vi "Init.vi"(8 "error in (no error)":errorcluster, 11 "DtoA in":refnum<class "Wavepond.lvclass">) -> (0 "error out":errorcluster, 3 "DtoA out":refnum<class "Wavepond.lvclass">)   [LabVIEW 2015, in "Wavepond.lvclass"]
uses:
  Wavepond.lvclass
  External Clock.lvclass
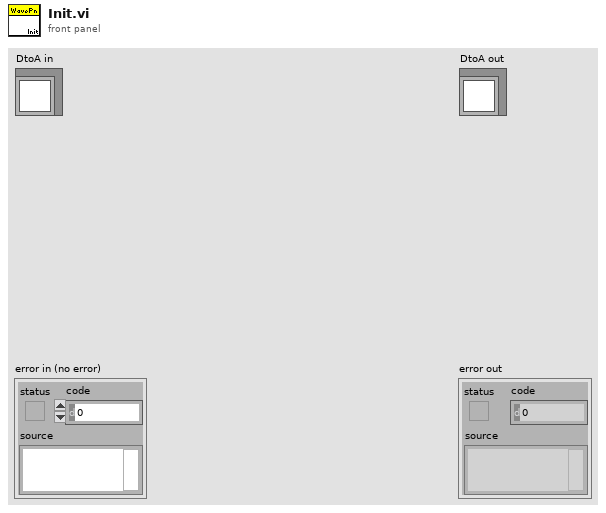
[diagram p1: front panel]
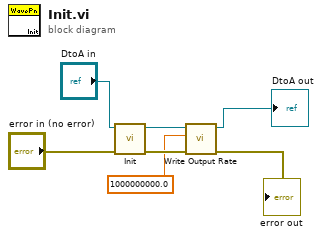
[diagram p0: block diagram]
diagram:
  n1 = call-parent "Init.vi"("error in (no error)"="error in (no error)", "DtoA in"="DtoA in") -> ("error out"=w4:errorcluster, "DtoA out"=w5:refnum<class "Wavepond.lvclass">)  [unwired: 8 in]
  n2 = call-dynamic "Write Output Rate.vi"("error in (no error)"=w4, "Output Rate"=1000000000.0, "External Clock in"=w5) -> ("error out"=→"error out":errorcluster, "External Clock out"=→"DtoA out":refnum<class "Wavepond.lvclass">)  [unwired: 7 in]
